vi "InitTestcaseListCtrl.vi"(10 "clear column":u16[](array[numeric]), 11 "ArrayRef in":refnum<vi>) -> (3 "ArrayRef out":refnum<vi>)   [LabVIEW 2018, in "Library-Ctrl.lvlib"]
uses:
  Library-Ctrl.lvlib
  <vilib>/Utility/miscctls.llb/LVRowAndColumnUnsignedTypeDef.ctl
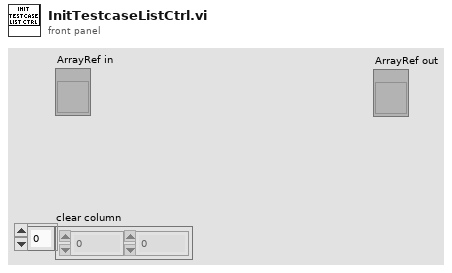
[diagram p1: front panel]
types:
  T1 = typedef "LVRowAndColumnUnsignedTypeDef.ctl" = cluster{"Row":u32, "Column":u32}
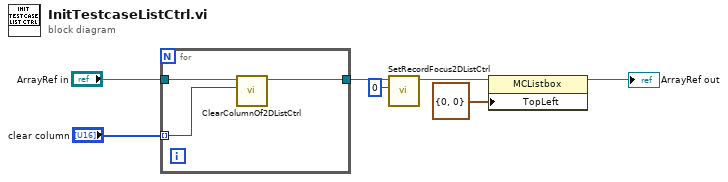
[diagram p0: block diagram]
diagram:
  n1 = for {
    tunnel: "clear column" -> [w9] mode=indexing
    tunnel: "ArrayRef in" -> [w10]
    tunnel: [w8] -> w1
    n2 = call "ClearColumnOf2DListCtrl.vi"("column"=w9, "ArrayRef in"=w10) -> ("ArrayRef out"=w8:refnum<vi>)  [unwired: 9 in]
  }
  n3 = call "SetRecordFocus2DListCtrl.vi"("index"=u16 0, "multiple list in"=w1) -> ("multiple list out"=w6:refnum<vi>)  [unwired: 9 in]
  n4 = property class="MCListbox"(reference=w6, "TopLeft"=T1 {"Row"=0, "Column"=0} ("왼쪽 위에 보이는 셀")) -> (reference out=→"ArrayRef out":refnum<vi>)  [unwired: 1 in, 1 out]
